vi "Pausable Timer Using Express VI.vi"() -> ()   [LabVIEW 2015]
panel:
  out "Elapsed Time (s) 2":dbl caption="Elapsed Time (s)"
  out "Time has Elapsed":bool
  out "Elapsed Time (s)":i32
  in  "Timer":i32=10
  in  "Stop":bool
  in  "Pause":bool
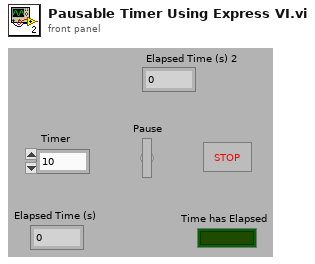
[diagram p1: front panel]
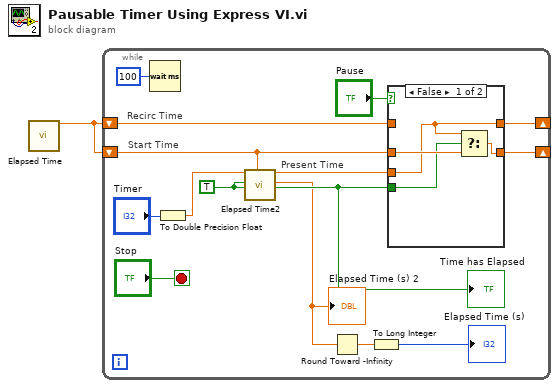
[diagram p0: block diagram]
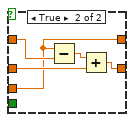
[diagram p2: hidden frame]
diagram:
  n1 = call "Elapsed Time"() -> ("Present (s)"=w1:dbl)  [unwired: 5 in, 14 out]
  n2 = while {
    shift-right: [w12] -> _
    shift-left: w1 -> [w13]
    shift-right: [w11] -> _
    shift-left: w1 -> [w5]
    stop <- "Stop" stop-if-true
    w9 = TRUE ("Reset")
    # "Present Time"
    # "Start Time"
    # "Recirc Time"
    n3 = Wait (ms)(milliseconds to wait=u32 100) -> ()  [unwired: 1 out]
    n4 = To Double Precision Float(number="Timer") -> (double precision float=w10:dbl)
    n5 = call "Elapsed Time2"("Time Target (s)"=w10, "Reset"=w9, "Auto Reset"=w9, "Set Start Time (s)"=w5) -> ("Present (s)"=w7:dbl, "Elapsed Time (s)"=w4:dbl, "Time has Elapsed"=w6:bool)  [unwired: 1 in, 12 out]
    "Time has Elapsed" <- w6
    "Elapsed Time (s) 2" <- w4
    n6 = Round Toward -Infinity(1:w4) -> (0:w3:dbl)
    n7 = To Long Integer(number=w3) -> (32bit integer=→"Elapsed Time (s)":i32)
    n8 = case shown="False" "Pause" {
      tunnel: w13 -> [_ w24]
      tunnel: w5 -> [w19 w25]
      tunnel: [w17 w21] -> w12
      tunnel: [w20 w22] -> w11
      tunnel: w7 -> [w17 w21]
      tunnel: w6 -> [w18 _]
      frame False {
        n9 = Select(t=w17, s=w18, f=w19) -> (s? t:f=w20:dbl)
      }
      frame True {
        n10 = Subtract(x=w21, y=w24) -> (x-y=w23:dbl)
        n11 = Add(x=w23, y=w25) -> (x+y=w22:dbl)
      }
    }
  }
